vi "Get Result.vi"(6 "Last request":bool, 8 "error in (no error)":errorcluster, 11 "Instrument Recorder in":refnum<class "Spectrum Recorder too.lvclass">) -> (0 "error out":errorcluster, 2 "Result":refnum<class "Acquired Result.lvclass">, 3 "Instrument Recorder out":refnum<class "Spectrum Recorder too.lvclass">)   [LabVIEW 2016, in "Spectrum Recorder too.lvclass"]
uses:
  Spectrum Recorder too.lvclass
  Results/Acquired Result/Acquired Result.lvclass
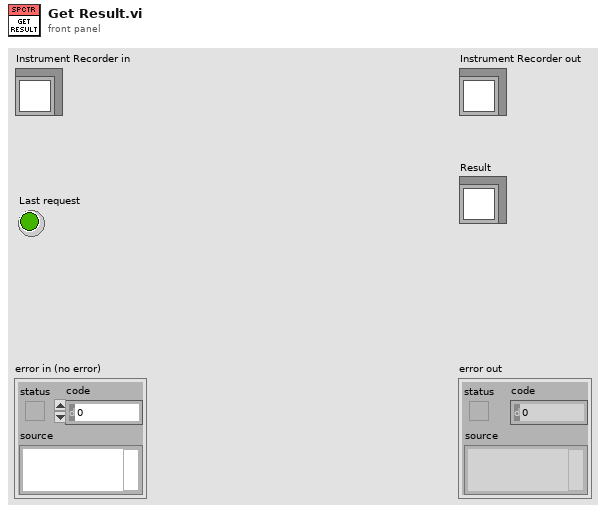
[diagram p1: front panel]
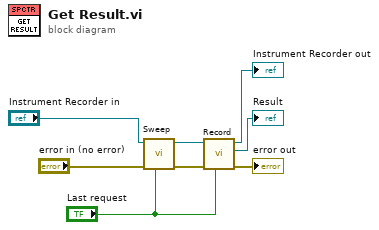
[diagram p0: block diagram]
diagram:
  n1 = call-dynamic "Sweep.vi"("Last request"="Last request", "error in (no error)"="error in (no error)", "Spectrum Recorder in"="Instrument Recorder in") -> ("error out"=w8:errorcluster, "Spectrum Recorder out"=w7:refnum<class "Spectrum Recorder too.lvclass">)  [unwired: 7 in]
  n2 = call-dynamic "Record.vi"("Last request"="Last request", "error in (no error)"=w8, "Spectrum Recorder in"=w7) -> ("error out"=→"error out":errorcluster, "Result"=→"Result":refnum<class "Acquired Result.lvclass">, "Spectrum Recorder out"=→"Instrument Recorder out":refnum<class "Spectrum Recorder too.lvclass">)  [unwired: 6 in]
